vi "String array to string.vi"(10 "delimiter (\\)":string="\\", 11 "Array":string[](array[string])) -> (3 "String":string)   [LabVIEW 2020, in "Blue Tree Map OpenSource.lvlib"]
uses:
  Blue Tree Map OpenSource.lvlib
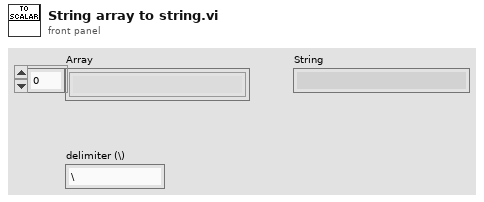
[diagram p1: front panel]
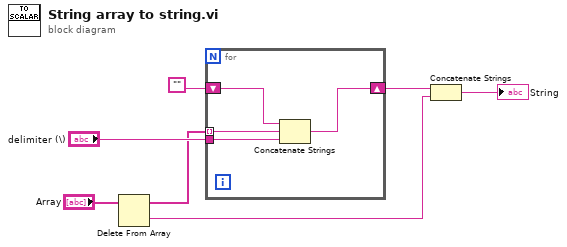
[diagram p0: block diagram]
diagram:
  n1 = Delete From Array(array="Array") -> (deleted portion=w2:string, array with subset deleted=w3:string[])  [unwired: 2 in]
  n2 = for {
    tunnel: w3 -> [w11] mode=indexing
    tunnel: "delimiter (\\)" -> [w8]
    shift-right: [w10] -> w5
    shift-left: "" -> [w9]
    n3 = Concatenate Strings(w9, w11, w8) -> (w10:string)
  }
  n4 = Concatenate Strings(w5, w2) -> (→"String":string)
